vi "PixyCamI2C.vi"(10 "Device Address":u8, 11 "I2C Bus":T1=enum."Invalid") -> ()   [LabVIEW 2017]
doc: "This VI reads the bolcks identified by a PixyCam. It is designed within the FRC framework and is expected to be run on a RoboRIO using the SPI ports.\nThe slave select pins are used so several PixyCam can be used. \nRefer to http://cmucam.org/projects/cmucam5/wiki/Porting_Guide for wiring and code explanation\nUse PixyMon to define the protocol and signatures\n\n(c)2017 PY Le Bas"
uses:
  <vilib>/Rock Robotics/SystemInterfaces/i2clib/i2c_bus.ctl
  Robot Global Data.vi
  <vilib>/Rock Robotics/Network Tables/NT Write Number.vi
panel:
  out "Blocks":T2(array[cluster])
  out "last frame data":u16[](array[numeric]) format="%.0x"
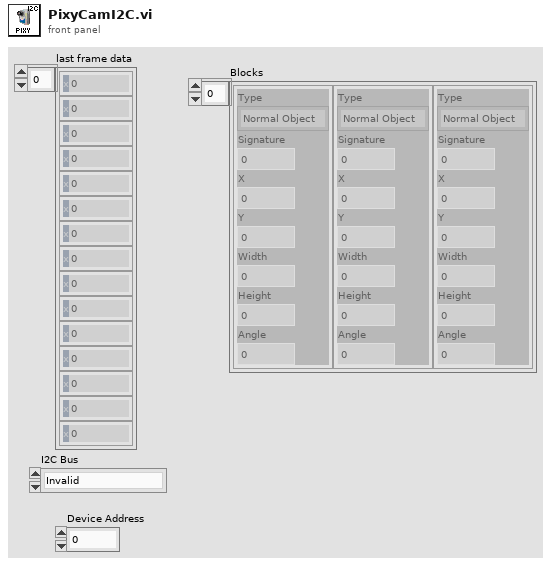
[diagram p1: front panel]
types:
  T1 = typedef "i2c_bus.ctl" = enum16{"I2C On-Board", "I2C MXP", "Invalid"}
  T2 = cluster{"Type":enum16{"Normal Object", "Color Object"}, "Signature":u16, "X":u16, "Y":u16, "Width":u16, "Height":u16, "Angle":u16}[]
  T3 = typedef "WPI_I2CDevRef.ctl" = cluster{"DevStatus":errorcluster, "Device Address":u8, "Handle":i32, "I2C Bus":T1}
  T4 = cluster{"Type":enum16{"Normal Object", "Color Object"}, "Signature":u16, "X":u16, "Y":u16, "Width":u16, "Height":u16, "Angle":u16}
  T5 = cluster{"[0]":u16, "[1]":u16, "[2]":u16, "[3]":u16, "[4]":u16, "[5]":u16, "[6]":u16}
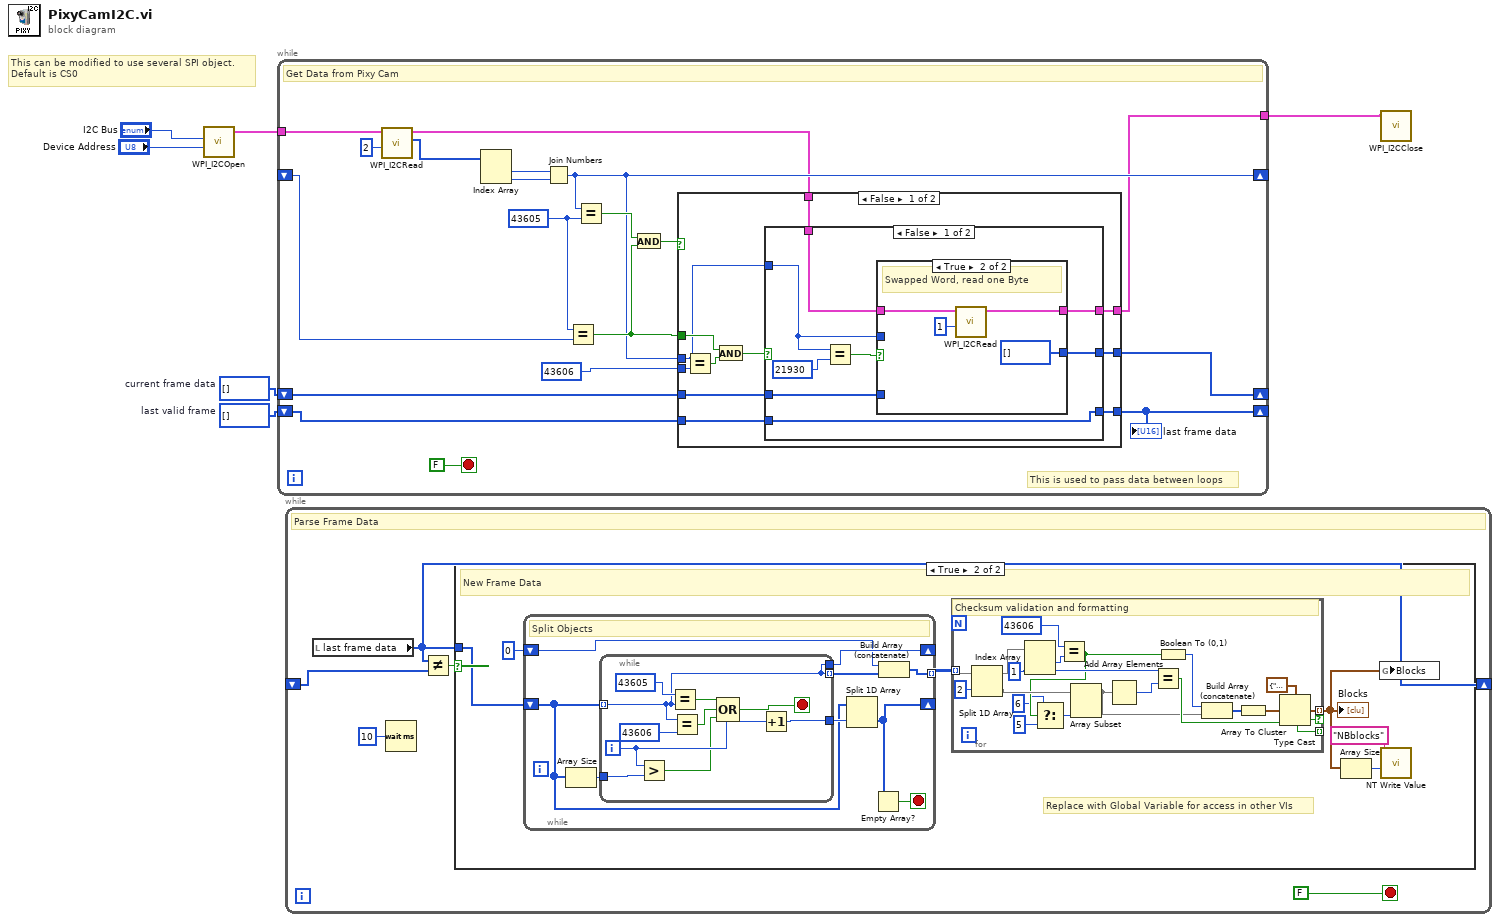
[diagram p0: block diagram]
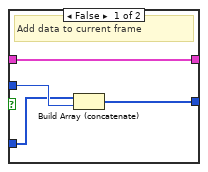
[diagram p3: hidden frame]
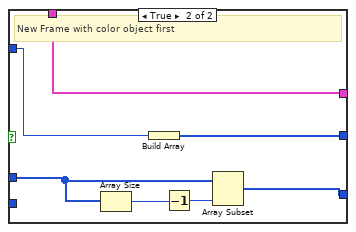
[diagram p4: hidden frame]
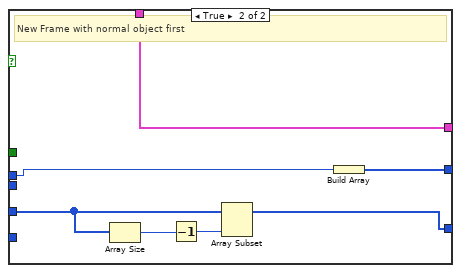
[diagram p5: hidden frame]
diagram:
  w5 = u16[] []  # current frame data
  w6 = u16[] []  # last valid frame
  # "This can be modified to use several SPI object.\nDefault is CS0"
  n1 = call <vilib>:"WPI_I2COpen.vi"("Device Address"="Device Address", "I2C Bus"="I2C Bus") -> ("I2CDevRef"=w4:T3)  [unwired: 8 in, 1 out]
  n2 = while {
    tunnel: w4 -> [w25]
    tunnel: [w14] -> w1
    shift-right: [w16] -> _
    shift-left: _ -> [w21]
    shift-right: [w12] -> _
    shift-left: w5 -> [w13]
    shift-right: [w11] -> _
    shift-left: w6 -> [w10]
    stop <- FALSE stop-if-true
    w9 = u16 43605
    # "This is used to pass data between loops"
    # "Get Data from Pixy Cam"
    n3 = call <vilib>:"WPI_I2CRead.vi"("I2CBytesToRead"=u8 2, "I2CDevRef"=w25) -> ("Data Out"=w24:u8[], "I2CDevRef"=w15:T3)  [unwired: 7 in, 1 out]
    n4 = Index Array(array=w24) -> (element #1=w23:u8, element #2=w22:u8)  [unwired: 2 in]
    n5 = Join Numbers(hi=w23, lo=w22) -> ((hi.lo)=w16:u16)
    n6 = Equal?(x=w9, y=w21) -> (x = y?=w18:bool)
    n7 = Equal?(x=w16, y=w9) -> (x = y?=w19:bool)
    n8 = And(x=w19, y=w18) -> (x .and. y?=w20:bool)
    n9 = case shown="False" w20 {
      tunnel: w18 -> [w36 _]
      tunnel: w16 -> [w26 w60]
      tunnel: u16 43606 -> [w34 _]
      tunnel: w15 -> [w32 w66]
      tunnel: [w31 w66] -> w14
      tunnel: w13 -> [w30 w63]
      tunnel: [w29 w61] -> w12
      tunnel: [w28 w65] -> w11
      tunnel: w10 -> [w27 _]
      frame False {
        n10 = Equal?(x=w26, y=w34) -> (x = y?=w35:bool)
        n11 = And(x=w36, y=w35) -> (x .and. y?=w33:bool)
        n12 = case shown="False" w33 {
          tunnel: w26 -> [w40 w54]
          tunnel: w32 -> [w43 w59]
          tunnel: [w42 w59] -> w31
          tunnel: w30 -> [w39 w56]
          tunnel: [w38 w53] -> w29
          tunnel: [w37 w55] -> w28
          tunnel: w27 -> [w37 _]
          frame False {
            n13 = Equal?(x=w40, y=u16 21930) -> (x = y?=w41:bool)
            n14 = case shown="True" w41 {
              tunnel: w43 -> [w48 w50]
              tunnel: [w48 w49] -> w42
              tunnel: w40 -> [w47 _]
              tunnel: w39 -> [w46 _]
              tunnel: [w45 u16[] []] -> w38
              frame False {
                # "Add data to current frame"
                n15 = Build Array (concatenate)(w46, w47) -> (w45:u16[])
              }
              frame True {
                # "Swapped Word, read one Byte"
                n16 = call <vilib>:"WPI_I2CRead.vi"("I2CBytesToRead"=u8 1, "I2CDevRef"=w50) -> ("I2CDevRef"=w49:T3)  [unwired: 7 in, 2 out]
              }
            }
          }
          frame True {
            # "New Frame with color object first"
            n17 = Array Size(array=w56) -> (size(s)=w58:i32)
            n18 = Build Array(w54) -> (w53:u16[])
            n19 = Decrement(x=w58) -> (x-1=w57:i32)
            n20 = Array Subset(array=w56, length=w57) -> (w55:u16[])  [unwired: 1 in]
          }
        }
      }
      frame True {
        # "New Frame with normal object first"
        n21 = Array Size(array=w63) -> (size(s)=w64:i32)
        n22 = Decrement(x=w64) -> (x-1=w62:i32)
        n23 = Array Subset(array=w63, length=w62) -> (w65:u16[])  [unwired: 1 in]
        n24 = Build Array(w60) -> (w61:u16[])
      }
    }
    "last frame data" <- w11
  }
  n25 = while {
    shift-right: [w69] -> _
    shift-left: _ -> [w71]
    stop <- FALSE stop-if-true
    # "Parse Frame Data"
    n26 = local read "last frame data"() -> (w69:u16[])
    n27 = Wait (ms)(milliseconds to wait=u32 10) -> ()  [unwired: 1 out]
    n28 = Not Equal?(x=w69, y=w71) -> (x != y?=w70:bool)
    n29 = case shown="True" w70 {
      tunnel: w69 -> [_ w76]
      frame False {
        # "Same Frame"
      }
      frame True {
        # "Replace with Global Variable for access in other VIs"
        # "New Frame Data"
        n30 = while {
          shift-right: [w104] -> _
          shift-left: w76 -> [w102]
          tunnel: [w100] -> w75 mode=indexing
          shift-right: [w99] -> _
          shift-left: u16 0 -> [w98]
          stop <- w103 stop-if-true
          # "Split Objects"
          n31 = Array Size(array=w102) -> (size(s)=w101:i32)
          n32 = while {
            tunnel: w102 -> [w107] mode=indexing
            tunnel: [w107] -> w106 mode=indexing
            tunnel: [w112] -> w105
            tunnel: w101 -> [w110]
            tunnel: [w107] -> w99
            i -> [w109]
            stop <- w113 stop-if-true
            n33 = Greater?(x=w109, y=w110) -> (0:w108:bool)
            n34 = Equal?(x=u16 43605, y=w107) -> (x = y?=w115:bool)
            n35 = Equal?(x=w107, y=u16 43606) -> (x = y?=w114:bool)
            n36 = Compound Arithmetic op=OR(w115, w114, w108) -> (w113:bool)
            n37 = Increment(x=w109) -> (x+1=w112:i32)
          }
          n38 = Split 1D Array(array=w102, index=w105) -> (second subarray=w104:u16[])  [unwired: 1 out]
          n39 = Empty Array?(array=w104) -> (empty?=w103:bool)
          n40 = Build Array (concatenate)(w98, w106) -> (w100:u16[])
        }
        n41 = for {
          tunnel: w75 -> [w97] mode=indexing
          tunnel: [w86] -> w72 mode=indexing if=w84
          tunnel: [w84] -> _ mode=indexing
          # "Checksum validation and formatting"
          n42 = Split 1D Array(array=w97, index=2) -> (first subarray=w95:u16[], second subarray=w83:u16[])
          n43 = Index Array(array=w95, index #2=1 ("index")) -> (element #1=w89:u16, element #2=w94:u16)  [unwired: 1 in]
          n44 = Equal?(x=u16 43606, y=w89) -> (x = y?=w80:bool)
          n45 = Select(t=6 ("index"), s=w80, f=5 ("index")) -> (s? t:f=w81:i32)
          n46 = Array Subset(array=w83, length=w81) -> (w82:u16[])  [unwired: 1 in]
          n47 = Add Array Elements(numeric array=w82) -> (sum=w93:u16)
          n48 = Equal?(x=w94, y=w93) -> (x = y?=w84:bool)
          n49 = Boolean To (0,1)(Boolean=w80) -> (0, 1=w87:i16)
          n50 = Build Array (concatenate)(w87, w82) -> (w90:u16[])
          n51 = Array To Cluster(array=w90) -> (cluster=w91:T5)
          n52 = Type Cast(type=T4 {"Type"=enum."Color Object", "Signature"=1, "X"=100, "Y"=36, "Width"=50, "Height"=48, "Angle"=0} ("Blocks"), x=w91) -> (*(type *) &x=w86:T4)
        }
        "Blocks" <- w72
        n53 = Array Size(array=w72) -> (size(s)=w73:i32)
        n54 = global write "Robot Global Data.vi" "Blocks"(w72) -> ()
        n55 = call-poly <vilib>:"NT Write Value.vi"("Numeric"=w73, "Name"="NBblocks") -> ()  [unwired: 9 in, 1 out]
      }
    }
  }
  n56 = call <vilib>:"WPI_I2CClose.vi"("I2CDevRef"=w1) -> ()  [unwired: 10 in, 1 out]
